vi "List.vi"(7 "Qualified Name":string, 8 "error in (no error)":errorcluster, 11 "ConfigManager in":refnum<class "ConfigManager.lvclass">) -> (0 "error out":errorcluster, 2 "Keys":string[](array[string]), 3 "ConfigManager out":refnum<class "ConfigManager.lvclass">)   [LabVIEW 2013, in "SMOConfig.lvlib" / "ConfigManager.lvclass"]
uses:
  ConfigManager.lvclass
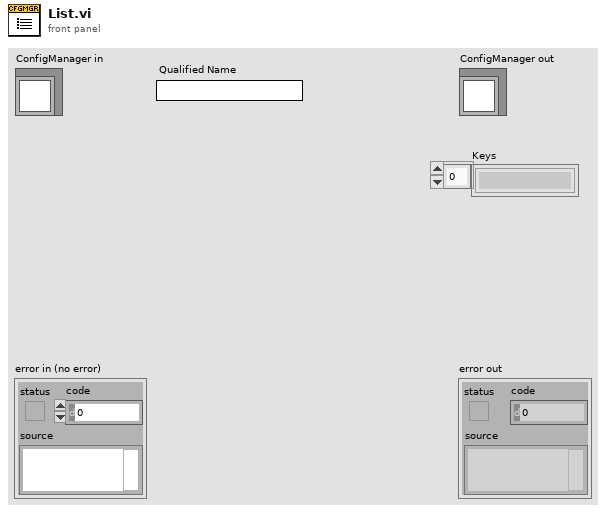
[diagram p1: front panel]
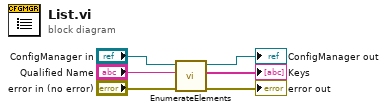
[diagram p0: block diagram]
diagram:
  n1 = call-dynamic "EnumerateElements.vi"("error in (no error)"="error in (no error)", "Qualified Name"="Qualified Name", "ConfigManager in"="ConfigManager in") -> ("error out"=→"error out":errorcluster, "keys"=→"Keys":string[], "ConfigManager out"=→"ConfigManager out":refnum<class "ConfigManager.lvclass">)  [unwired: 6 in]
